vi "VCI_BOARD_INFO1_1_CONVERT.vi"(1 "VCI_BOARD_INFO1_1":T2) -> (0 "VCI_BOARD_INFO1":T1)   [LabVIEW 2018, in "ControlCan.lvlib"]
uses:
  ControlCan.lvlib
  VCI_BOARD_INFO1_1.ctl
  VCI_BOARD_INFO1.ctl
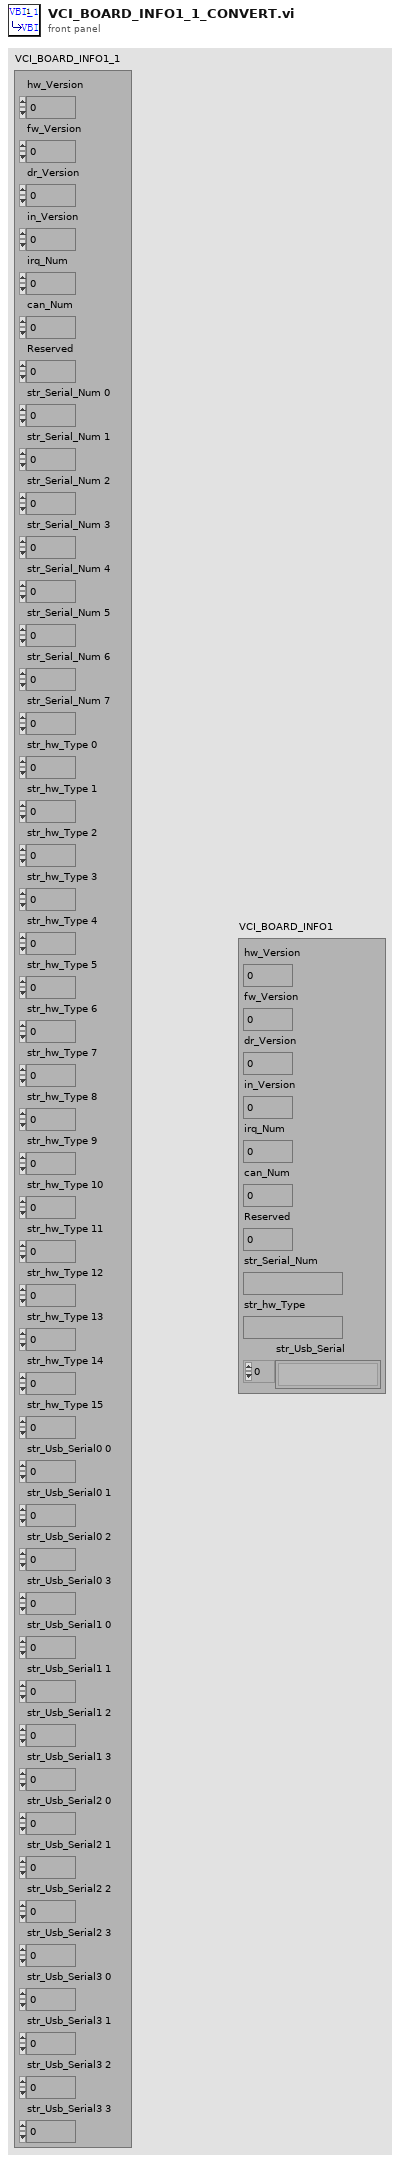
[diagram p1: front panel]
types:
  T1 = typedef "ControlCAN.lvlib/VCI_BOARD_INFO1.ctl" = cluster{"hw_Version":u16, "fw_Version":u16, "dr_Version":u16, "in_Version":u16, "irq_Num":u16, "can_Num":u8, "Reserved":u8, "str_Serial_Num":string, "str_hw_Type":string, "str_Usb_Serial":string[]}
  T2 = typedef "ControlCAN.lvlib/VCI_BOARD_INFO1_1.ctl" = cluster{"hw_Version":u16, "fw_Version":u16, "dr_Version":u16, "in_Version":u16, "irq_Num":u16, "can_Num":u8, "Reserved":u8, "str_Serial_Num 0":u8, "str_Serial_Num 1":u8, "str_Serial_Num 2":u8, "str_Serial_Num 3":u8, "str_Serial_Num 4":u8, "str_Serial_Num 5":u8, "str_Serial_Num 6":u8, "str_Serial_Num 7":u8, "str_hw_Type 0":u8, "str_hw_Type 1":u8, "str_hw_Type 2":u8, "str_hw_Type 3":u8, "str_hw_Type 4":u8, "str_hw_Type 5":u8, "str_hw_Type 6":u8, "str_hw_Type 7":u8, "str_hw_Type 8":u8, "str_hw_Type 9":u8, "str_hw_Type 10":u8, "str_hw_Type 11":u8, "str_hw_Type 12":u8, "str_hw_Type 13":u8, "str_hw_Type 14":u8, "str_hw_Type 15":u8, "str_Usb_Serial0 0":u8, "str_Usb_Serial0 1":u8, "str_Usb_Serial0 2":u8, "str_Usb_Serial0 3":u8, "str_Usb_Serial1 0":u8, "str_Usb_Serial1 1":u8, "str_Usb_Serial1 2":u8, "str_Usb_Serial1 3":u8, "str_Usb_Serial2 0":u8, "str_Usb_Serial2 1":u8, "str_Usb_Serial2 2":u8, "str_Usb_Serial2 3":u8, "str_Usb_Serial3 0":u8, "str_Usb_Serial3 1":u8, "str_Usb_Serial3 2":u8, "str_Usb_Serial3 3":u8}
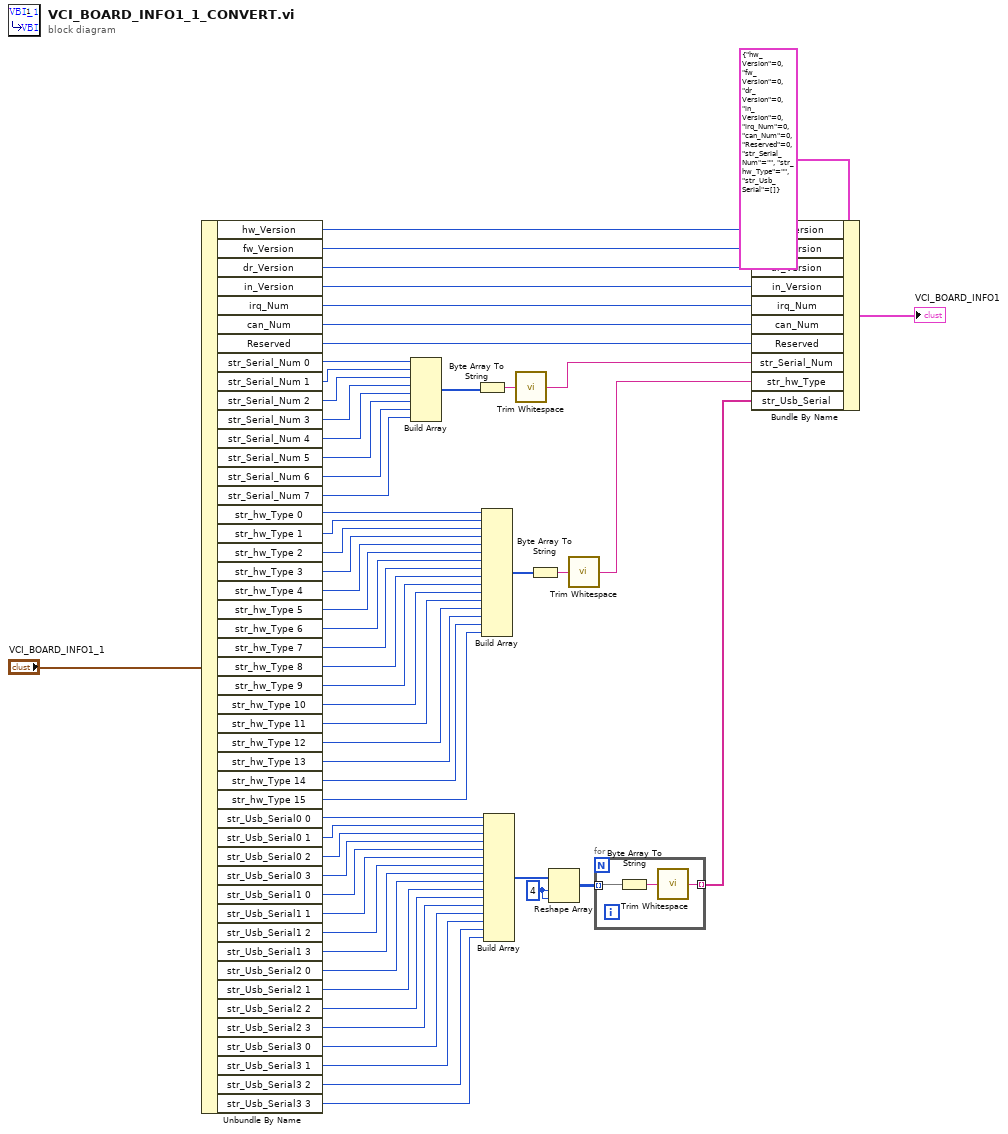
[diagram p0: block diagram]
diagram:
  w4 = 4 ("维数大小")
  n1 = Unbundle By Name("VCI_BOARD_INFO1_1") -> ("hw_Version"=w57:u16, "fw_Version"=w56:u16, "dr_Version"=w55:u16, "in_Version"=w54:u16, "irq_Num"=w53:u16, "can_Num"=w52:u8, "Reserved"=w51:u8, "str_Serial_Num 0"=w50:u8, "str_Serial_Num 1"=w49:u8, "str_Serial_Num 2"=w48:u8, "str_Serial_Num 3"=w47:u8, "str_Serial_Num 4"=w46:u8, "str_Serial_Num 5"=w45:u8, "str_Serial_Num 6"=w44:u8, "str_Serial_Num 7"=w43:u8, "str_hw_Type 0"=w40:u8, "str_hw_Type 1"=w39:u8, "str_hw_Type 2"=w38:u8, "str_hw_Type 3"=w37:u8, "str_hw_Type 4"=w36:u8, "str_hw_Type 5"=w35:u8, "str_hw_Type 6"=w34:u8, "str_hw_Type 7"=w33:u8, "str_hw_Type 8"=w32:u8, "str_hw_Type 9"=w31:u8, "str_hw_Type 10"=w30:u8, "str_hw_Type 11"=w29:u8, "str_hw_Type 12"=w28:u8, "str_hw_Type 13"=w27:u8, "str_hw_Type 14"=w26:u8, "str_hw_Type 15"=w25:u8, "str_Usb_Serial0 0"=w21:u8, "str_Usb_Serial0 1"=w20:u8, "str_Usb_Serial0 2"=w19:u8, "str_Usb_Serial0 3"=w18:u8, "str_Usb_Serial1 0"=w17:u8, "str_Usb_Serial1 1"=w16:u8, "str_Usb_Serial1 2"=w15:u8, "str_Usb_Serial1 3"=w14:u8, "str_Usb_Serial2 0"=w13:u8, "str_Usb_Serial2 1"=w12:u8, "str_Usb_Serial2 2"=w11:u8, "str_Usb_Serial2 3"=w10:u8, "str_Usb_Serial3 0"=w9:u8, "str_Usb_Serial3 1"=w8:u8, "str_Usb_Serial3 2"=w7:u8, "str_Usb_Serial3 3"=w6:u8)
  n2 = Build Array(w50, w49, w48, w47, w46, w45, w44, w43) -> (w42:u8[])
  n3 = Byte Array To String(unsigned byte array=w42) -> (string=w60:string)
  n4 = Build Array(w40, w39, w38, w37, w36, w35, w34, w33, w32, w31, w30, w29, w28, w27, w26, w25) -> (w23:u8[])
  n5 = Build Array(w21, w20, w19, w18, w17, w16, w15, w14, w13, w12, w11, w10, w9, w8, w7, w6) -> (w5:u8[])
  n6 = call <vilib>:"Trim Whitespace.vi"("string"=w60) -> ("trimmed string"=w41:string)  [unwired: 1 in]
  n7 = Byte Array To String(unsigned byte array=w23) -> (string=w24:string)
  n8 = Reshape Array(w5, w4, w4) -> (w3:u8[][])
  n9 = call <vilib>:"Trim Whitespace.vi"("string"=w24) -> ("trimmed string"=w22:string)  [unwired: 1 in]
  n10 = for {
    tunnel: w3 -> [w62] mode=indexing
    tunnel: [w61] -> w2 mode=indexing
    n11 = Byte Array To String(unsigned byte array=w62) -> (string=w63:string)
    n12 = call <vilib>:"Trim Whitespace.vi"("string"=w63) -> ("trimmed string"=w61:string)  [unwired: 1 in]
  }
  n13 = Bundle By Name(cluster=T1 {"hw_Version"=0, "fw_Version"=0, "dr_Version"=0, "in_Version"=0, "irq_Num"=0, "can_Num"=0, "Reserved"=0, "str_Serial_Num"="", "str_hw_Type"="", "str_Usb_Serial"=[]} ("VCI_BOARD_INFO1"), "hw_Version"=w57, "fw_Version"=w56, "dr_Version"=w55, "in_Version"=w54, "irq_Num"=w53, "can_Num"=w52, "Reserved"=w51, "str_Serial_Num"=w41, "str_hw_Type"=w22, "str_Usb_Serial"=w2) -> (→"VCI_BOARD_INFO1":T1)
